vi "Setting.vi"() -> ()   [LabVIEW 2015]
panel:
  in  "設備試運轉":bool
  in  "異常履歷":bool
  in  "I/O":bool
  in  "手動":bool
  in  "教導":bool
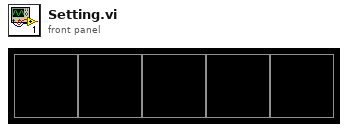
[diagram p1: front panel]
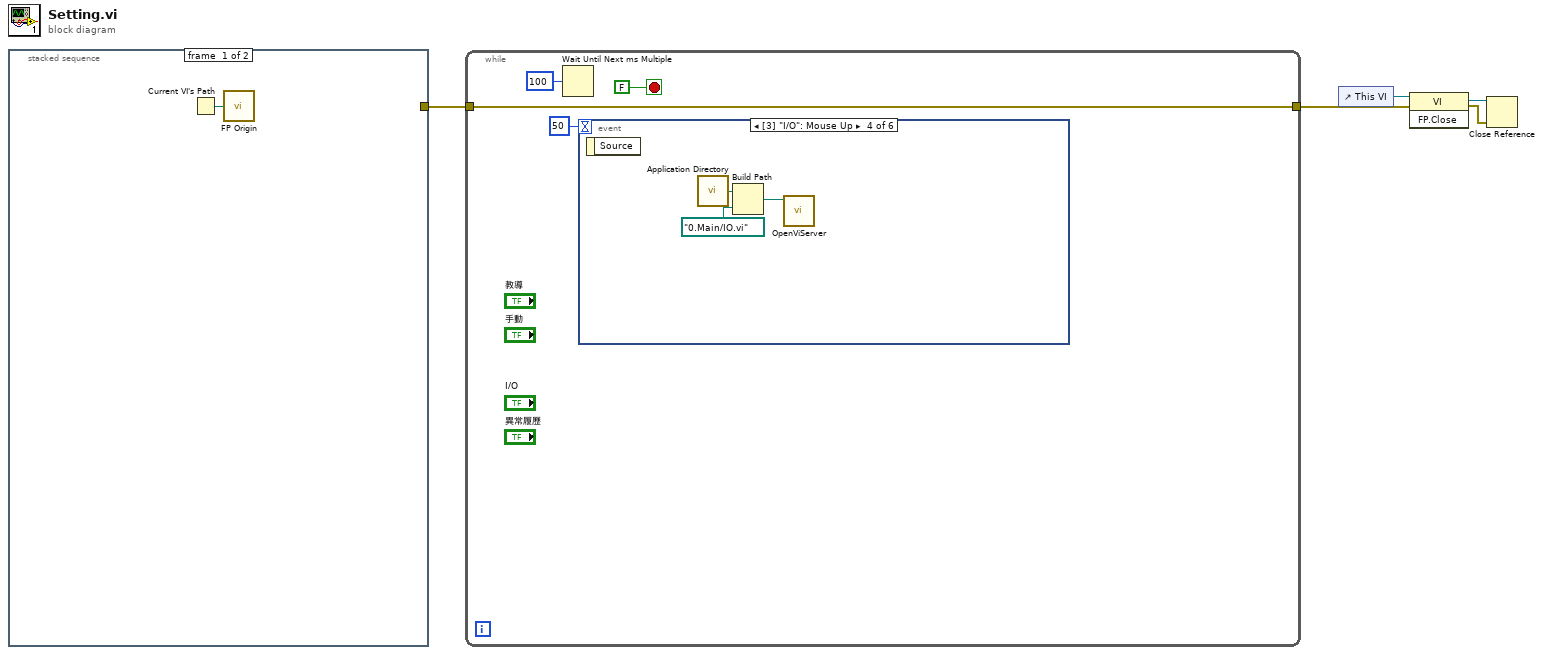
[diagram p0: block diagram]
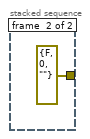
[diagram p2: hidden frame]
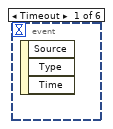
[diagram p3: hidden frame]
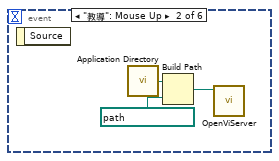
[diagram p4: hidden frame]
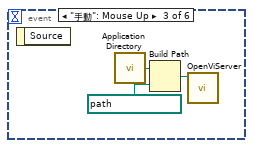
[diagram p5: hidden frame]
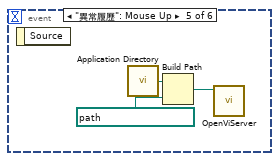
[diagram p6: hidden frame]
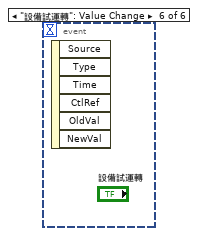
[diagram p7: hidden frame]
diagram:
  n1 = stacked-sequence {
    tunnel: [_ errorcluster {"status"=FALSE, "code"=0, "source"=""} ("error out")] -> w1
    frame #0 {
      n2 = Current VI's Path() -> (path=w6:path)
      n3 = call "FP Origin.vi"("vi path"=w6) -> ()  [unwired: 1 out]
    }
    frame #1 {
    }
  }
  n4 = while {
    tunnel: w1 -> [w9]
    tunnel: [w9] -> w5
    stop <- FALSE stop-if-true
    n5 = Wait Until Next ms Multiple(millisecond multiple=u32 100) -> ()  [unwired: 1 out]
    n6 = event shown="[3] \"I/O\": Mouse Up" {
      selector: _ -> [_ _ _ _ _ _]
      dyn-events: _ -> [_ _ _ _ _ _]
      timeout: 50 -> [_ _ _ _ _ _]
      event Timeout {
        n7 = event-data() -> ()  [unwired: 1 in, 3 out]
      }
      event "教導": Mouse Up {
        n8 = event-data() -> ()  [unwired: 1 in, 1 out]
        n9 = call <vilib>:"Application Directory.vi"() -> ("Application Directory"=w14:path)
        n10 = Build Path(base path=w14, name or relative path=path "0.Main/教導.vi" ("vi path")) -> (appended path=w12:path)
        n11 = call "OpenViServer.vi"("vi path"=w12) -> ()  [unwired: 9 in, 2 out]
      }
      event "手動": Mouse Up {
        n12 = event-data() -> ()  [unwired: 1 in, 1 out]
        n13 = call <vilib>:"Application Directory.vi"() -> ("Application Directory"=w15:path)
        n14 = Build Path(base path=w15, name or relative path=path "0.Main/手動.vi" ("vi path")) -> (appended path=w17:path)
        n15 = call "OpenViServer.vi"("vi path"=w17) -> ()  [unwired: 9 in, 2 out]
      }
      event "I/O": Mouse Up {
        n16 = event-data() -> ()  [unwired: 1 in, 1 out]
        n17 = call <vilib>:"Application Directory.vi"() -> ("Application Directory"=w20:path)
        n18 = Build Path(base path=w20, name or relative path=path "0.Main/IO.vi" ("vi path")) -> (appended path=w18:path)
        n19 = call "OpenViServer.vi"("vi path"=w18) -> ()  [unwired: 9 in, 2 out]
      }
      event "異常履歷": Mouse Up {
        n20 = event-data() -> ()  [unwired: 1 in, 1 out]
        n21 = call <vilib>:"Application Directory.vi"() -> ("Application Directory"=w23:path)
        n22 = Build Path(base path=w23, name or relative path=path "0.Main/異常履歷.vi" ("vi path")) -> (appended path=w21:path)
        n23 = call "OpenViServer.vi"("vi path"=w21) -> ()  [unwired: 9 in, 2 out]
      }
      event "設備試運轉": Value Change {
        n24 = event-data() -> ()  [unwired: 1 in, 6 out]
      }
    }
  }
  n25 = control-ref of="This VI"() -> (w4:refnum<vi>)
  n26 = invoke class="VI" method="FP.Close"(reference=w4, error in=w5) -> (reference out=w3:refnum<vi>, error out=w2:errorcluster)  [unwired: 1 in, 1 out]
  n27 = Close Reference(reference=w3, error in (no error)=w2) -> ()  [unwired: 1 out]
